vi "Samples Elapsed.vi"(8 "error in (no error)":errorcluster, 9 "SE":u32, 10 "TC":u32, 11 "Present Terminal":u32) -> (0 "error out":errorcluster, 3 "Samples Elapsed":bool)   [LabVIEW 2019, in "Zen Analytics.lvlib" / "Zen Analytics.lvclass"]
uses:
  Zen Analytics.lvclass
panel:
  out "diff":u32
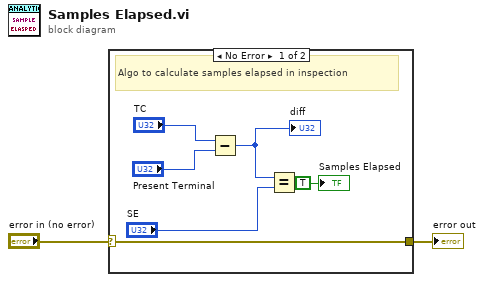
[diagram p0: block diagram]
diagram:
  n1 = case shown="No Error" "error in (no error)" {
    selector: "error in (no error)" -> [w8 w9]
    tunnel: [w8 w9] -> w1
    frame No Error {
      # "Algo to calculate samples elapsed in inspection"
      n2 = Subtract(x="TC", y="Present Terminal") -> (x-y=w5:u32)
      "diff" <- w5
      n3 = Equal?(x=w5, y="SE") -> ()  [unwired: 1 out]
      "Samples Elapsed" <- TRUE ("Samples Elapsed")
    }
    frame Error {
    }
  }
  "error out" <- w1
